vi "SerialPositionCalibration.vi"() -> ()   [LabVIEW 2017]
uses:
  <vilib>/Analysis/baseanly.llb/Mean (DBL).vi
  <vilib>/Instr/_visa.llb/VISA Configure Serial Port (Instr).vi
  <vilib>/express/express shared/transition.llb/Dynamic To Waveform Array.vi
  <vilib>/express/express signal manip/GetorSetDDTAttributes/Set DDT Attributes/SetT0.vi
  <vilib>/express/express shared/transition.llb/Waveform Array To Dynamic.vi
  <vilib>/express/express signal manip/GetorSetDDTAttributes/Set DDT Attributes/Set DDT Properties.xnode
  <vilib>/Analysis/NI_AALBase.lvlib
  <vilib>/Analysis/NI_AALPro.lvlib
panel:
  in  "Filename":path=path "Servo1PosCal.xlsx"
  out "PWM Array":dbl[](array[numeric])
  out "Angle vs PWM Quadratic Coefficients":dbl[](array[numeric])
  out "Angle vs PWM Linear Coefficients":dbl[](array[numeric])
  out "Angle vs PWM":cluster{dbl[], dbl[]}(graph)
  out "ADC vs  Angle Quadratic Coefficients":dbl[](array[numeric])
  out "ADC vs  Angle Linear Coefficients":dbl[](array[numeric])
  in  "Save Data":bool
  in  "Baud Rate":dbl=115200.0
  out "Angle Array":dbl[](array[numeric])
  out "ADC Value Array":dbl[](array[numeric])
  out "ADC Value vs Angle":cluster{dbl[], dbl[]}(graph)
  out "Average ADC Value":dbl format="%0.2f"
  out "Live ADC Value":cluster{i32, dbl, dbl[]}(graph)
  in  "Com Port":refnum<visa-resource-name>="ASRL1::INSTR"
  in  "Sample Frequency":dbl=200.0
  in  "Number of Samples":dbl=100.0
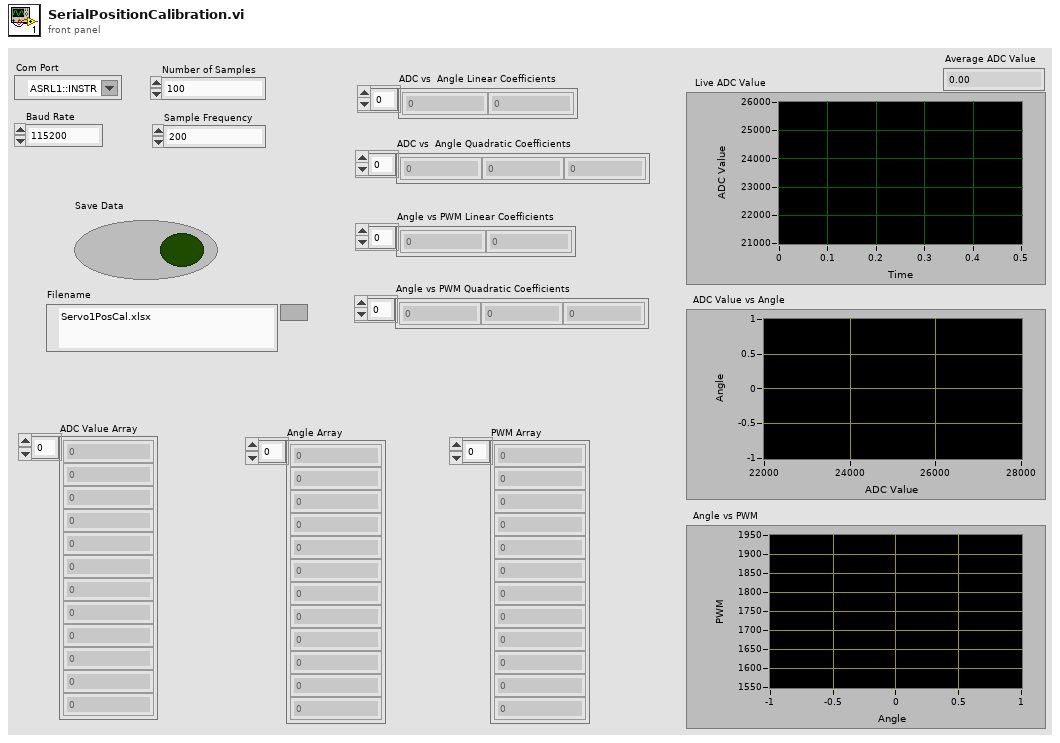
[diagram p1: front panel]
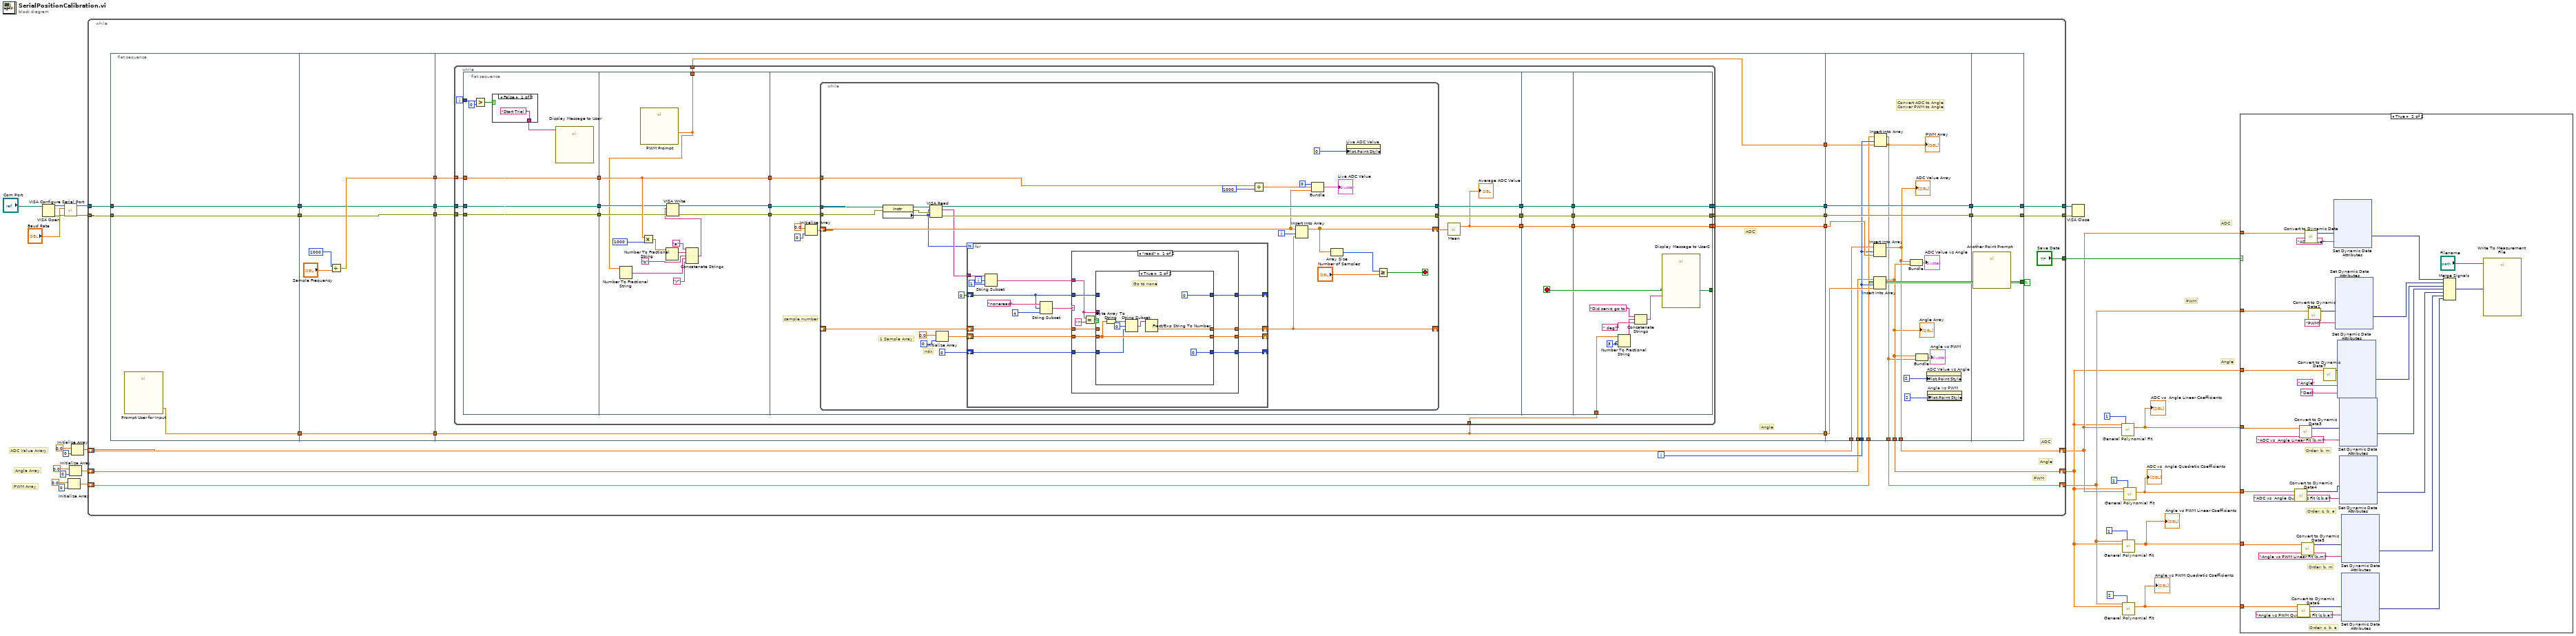
[diagram p0: block diagram]
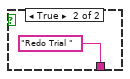
[diagram p3: hidden frame]
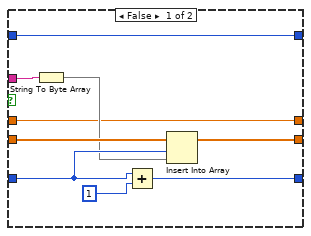
[diagram p4: hidden frame]
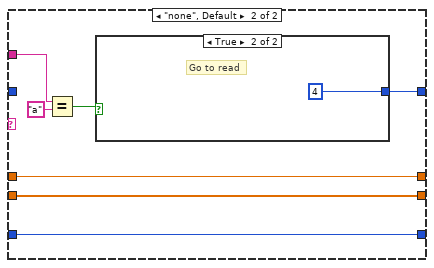
[diagram p5: hidden frame]
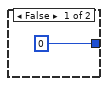
[diagram p6: hidden frame]
diagram:
  # "PWM Array"
  # "ADC"
  # "PWM"
  # "Angle"
  # "Angle Array"
  # "ADC Value Arrary"
  n1 = VISA Open(VISA resource name="Com Port") -> (VISA resource name=w28:refnum<visa-resource-name>, error out=w27:errorcluster)  [unwired: 4 in]
  n2 = call-poly "VISA Configure Serial Port"("VISA resource name"=w28, "baud rate (9600)"="Baud Rate", "error in (no error)"=w27) -> ("VISA resource name out"=w26:refnum<visa-resource-name>, "error out"=w25:errorcluster)  [unwired: 11 in]
  n3 = Initialize Array(0.0 ("element"), 0 ("dimension size")) -> (w4:dbl[])
  n4 = Initialize Array(0.0 ("element"), 0 ("dimension size")) -> (w17:dbl[])
  n5 = Initialize Array(0.0 ("element"), 0 ("dimension size")) -> (w18:dbl[])
  n6 = while {
    tunnel: w26 -> [w55]
    tunnel: w25 -> [w54]
    tunnel: [w52] -> w24
    tunnel: [w51] -> w23
    shift-right: [w32] -> w2
    shift-left: w18 -> [w35]
    shift-right: [w33] -> w1
    shift-left: w17 -> [w34]
    tunnel: ["Save Data"] -> w15
    shift-right: [w30] -> w3
    shift-left: w4 -> [w31]
    i -> [w40]
    stop <- w56 continue-if-true
    # "PWM"
    # "Angle"
    # "ADC"
    n7 = flat-sequence {
      tunnel: w54 -> [w58]
      tunnel: w55 -> [w59]
      tunnel: [w59] -> w49
      tunnel: [w58] -> w48
      tunnel: [w57] -> w46
      tunnel: [w60] -> w53
      tunnel: [w62] -> w50
      tunnel: w49 -> [w61]
      tunnel: w48 -> [w60]
      tunnel: [w64] -> w47
      tunnel: w46 -> [w64]
      tunnel: [w61] -> w45
      tunnel: w53 -> [w72]
      tunnel: [w68] -> w43
      tunnel: w50 -> [w71]
      tunnel: w47 -> [w67]
      tunnel: w45 -> [w73]
      tunnel: [w67] -> w39
      tunnel: [w70] -> w38
      tunnel: [w69] -> w37
      tunnel: [w66] -> w36
      tunnel: w43 -> [w236]
      tunnel: [w236] -> w42
      tunnel: [w235] -> w41
      tunnel: w40 -> [w228]
      tunnel: w39 -> [w232]
      tunnel: w38 -> [w229]
      tunnel: w37 -> [w235]
      tunnel: w36 -> [w227]
      tunnel: w35 -> [w226]
      tunnel: w34 -> [w225]
      tunnel: [w222] -> w33
      tunnel: [w224] -> w32
      tunnel: w31 -> [w223]
      tunnel: [w221] -> w30
      tunnel: [w239] -> w56
      tunnel: w42 -> [w238]
      tunnel: [w238] -> w52
      tunnel: [w237] -> w51
      tunnel: w41 -> [w237]
      frame #0 {
        n8 = call "Prompt User for Input"() -> ("Angle"=w57:dbl)  [unwired: 17 in, 2 out]
      }
      frame #1 {
        n9 = Divide(x=1000, y="Sample Frequency") -> (x/y=w62:dbl)
      }
      frame #2 {
        # "Angle"
        # "ADC"
        n10 = while {
          tunnel: w73 -> [w94]
          tunnel: w72 -> [w93]
          tunnel: [w92] -> w68
          tunnel: [w91] -> w69
          tunnel: w71 -> [w90]
          tunnel: [w89] -> w70
          tunnel: w67 -> [w81]
          tunnel: [w74] -> w66
          i -> [w82]
          stop <- w95 stop-if-true
          n11 = flat-sequence {
            tunnel: w90 -> [w100]
            tunnel: w93 -> [w101]
            tunnel: w94 -> [w102]
            tunnel: [w102] -> w80
            tunnel: [w101] -> w78
            tunnel: [w100] -> w77
            tunnel: w82 -> [w99]
            tunnel: w80 -> [w110]
            tunnel: [w108] -> w79
            tunnel: w78 -> [w109]
            tunnel: w77 -> [w111]
            tunnel: [w111] -> w76
            tunnel: [w107] -> w75
            tunnel: [w106] -> w74
            tunnel: [w126] -> w88
            tunnel: [w125] -> w86
            tunnel: [w119] -> w84
            tunnel: w79 -> [w128]
            tunnel: w76 -> [w124]
            tunnel: w75 -> [w127]
            tunnel: w88 -> [w210]
            tunnel: [w210] -> w87
            tunnel: w86 -> [w209]
            tunnel: [w209] -> w85
            tunnel: w84 -> [w208]
            tunnel: [w208] -> w83
            tunnel: [w217] -> w95
            tunnel: w87 -> [w220]
            tunnel: [w220] -> w92
            tunnel: [w219] -> w91
            tunnel: w85 -> [w219]
            tunnel: w83 -> [w218]
            tunnel: [w218] -> w89
            tunnel: w81 -> [w213]
            frame #0 {
              n12 = Greater?(x=w99, y=0) -> (0:w98:bool)
              n13 = case shown="False" w98 {
                tunnel: ["Start Trial " ("Message") "Redo Trial " ("Message")] -> w96
                frame False {
                }
                frame True {
                }
              }
              n14 = call "Display Message to User"("Message"=w96) -> ()  [unwired: 9 in, 2 out]
            }
            frame #1 {
              n15 = call "PWM Prompt"() -> ("PWM"=w106:dbl)  [unwired: 17 in, 2 out]
              n16 = Number To Fractional String(number=w106) -> (F-format string=w117:string)  [unwired: 3 in]
              n17 = Multiply(x=w111, y=1000) -> (x*y=w118:dbl)
              n18 = Number To Fractional String(number=w118) -> (F-format string=w116:string)  [unwired: 3 in]
              n19 = Concatenate Strings("a", w116, "b", w117, "\r") -> (w105:string)
              n20 = VISA Write(VISA resource name=w110, write buffer=w105, error in (no error)=w109) -> (VISA resource name out=w108:refnum<visa-resource-name>, error out=w107:errorcluster)  [unwired: 1 out]
            }
            frame #2 {
              # "sample number"
              n21 = Initialize Array(0.0, 0 ("dimension size")) -> (w123:dbl[])
              n22 = while {
                tunnel: w128 -> [w153]
                tunnel: w127 -> [w152]
                tunnel: [w151] -> w126
                tunnel: [w150] -> w125
                shift-right: [w138] -> _
                shift-left: _ -> [w144]
                tunnel: w124 -> [w133]
                shift-right: [w136] -> w120
                shift-left: w123 -> [w137]
                i -> [w139]
                stop <- w142 stop-if-true
                # "ndx"
                # "1 Sample Array"
                n23 = property class="Instr"(reference=w153, error in=w152) -> (reference out=w155:refnum<visa-resource-name>, error out=w154:errorcluster, "Serial Settings:Number of Bytes at Serial Port"=w130:u32)
                n24 = VISA Read(VISA resource name=w155, byte count=w130, error in (no error)=w154) -> (VISA resource name out=w151:refnum<visa-resource-name>, read buffer=w131:string, error out=w150:errorcluster)  [unwired: 1 out]
                n25 = Initialize Array(0.0 ("element"), 0 ("dimension size")) -> (w146:dbl[])
                n26 = for {
                  N: w130 -> [_]
                  tunnel: w131 -> [w169]
                  shift-right: [w165] -> _
                  shift-left: 0 -> [w164]
                  shift-right: [w160] -> _
                  shift-left: w146 -> [w161]
                  shift-right: [w159] -> _
                  shift-left: 0 ("dimension size") -> [w162]
                  shift-right: [w158] -> w138
                  shift-left: w144 -> [w157]
                  i -> [w168]
                  n27 = String Subset(string=w169, offset (0)=w168, length (rest)=1 ("length (rest)")) -> (substring=w163:string)
                  n28 = String Subset(string="noneread", offset (0)=w164, length (rest)=4 ("length (rest)")) -> (substring=w156:string)
                  n29 = case shown="\"read\"" w156 {
                    tunnel: [w181 w203] -> w165
                    tunnel: w164 -> [w180 _]
                    tunnel: w163 -> [w177 w202]
                    tunnel: w162 -> [w176 w199]
                    tunnel: w161 -> [w175 w200]
                    tunnel: [w174 w200] -> w160
                    tunnel: [w173 w199] -> w159
                    tunnel: [w172 w201] -> w158
                    tunnel: w157 -> [w171 w201]
                    frame "read" {
                      n30 = Equal?(x=w177, y="!") -> (x = y?=w179:bool)
                      n31 = case shown="True" w179 {
                        tunnel: [w190 0] -> w181
                        tunnel: w180 -> [w190 _]
                        tunnel: w177 -> [w187 _]
                        tunnel: w176 -> [w188 w192]
                        tunnel: w175 -> [w189 w195]
                        tunnel: [w185 w195] -> w174
                        tunnel: [w184 0] -> w173
                        tunnel: [w183 w197] -> w172
                        tunnel: w171 -> [w183 _]
                        frame False {
                          n32 = String To Byte Array(string=w187) -> (unsigned byte array=w186:u8[])
                          n33 = Add(x=w188, y=1 ("dimension size")) -> (x+y=w184:i32)
                          n34 = Insert Into Array(array=w189, index=w188, new element=w186) -> (w185:dbl[])
                        }
                        frame True {
                          # "Go to none"
                          n35 = Byte Array To String(unsigned byte array=w195) -> (string=w194:string)
                          n36 = String Subset(string=w194, offset (0)=0, length (rest)=w192) -> (substring=w193:string)
                          n37 = Fract/Exp String To Number(string=w193) -> (number=w197:dbl)  [unwired: 3 in, 1 out]
                        }
                      }
                    }
                    frame "none", Default {
                      n38 = Equal?(x=w202, y="a") -> (x = y?=w205:bool)
                      n39 = case shown="True" w205 {
                        tunnel: [0 4] -> w203
                        frame False {
                        }
                        frame True {
                          # "Go to read"
                        }
                      }
                    }
                  }
                }
                n40 = Divide(x=w133, y=1000) -> (x/y=w132:dbl)
                n41 = Insert Into Array(array=w137, index=w139, new element=w138) -> (w136:dbl[])
                n42 = Bundle(0, w132, w137) -> (→"Live ADC Value":cluster{i32, dbl, dbl[]})  [unwired: 1 in]
                n43 = Array Size(array=w136) -> (size(s)=w135:i32)
                n44 = property on="Live ADC Value" class="WFGraph (strict)"("Plot.Point Style"=u8 0) -> ()  [unwired: 2 in, 2 out]
                n45 = Greater Or Equal?(x=w135, y="Number of Samples") -> (x >= y?=w142:bool)
              }
              n46 = call-poly <vilib>:"Mean.vi"("X"=w120) -> ("mean"=w119:dbl)  [unwired: 1 out]
              "Average ADC Value" <- w119
            }
            frame #3 {
            }
            frame #4 {
              w211 = 3
              n47 = Number To Fractional String(number=w213, width (-)=w211, precision (6)=w211) -> (F-format string=w214:string)  [unwired: 1 in]
              n48 = Concatenate Strings("Did servo go to ", w214, " deg?") -> (w212:string)
              n49 = call "Display Message to User2"("Message"=w212) -> ("Yes"=w217:bool)  [unwired: 9 in, 1 out]
            }
          }
        }
      }
      frame #3 {
        # "Convert ADC to Angle\nConver PWM to Angle"
        n50 = Insert Into Array(array=w226, index=w228, new element=w229) -> (w224:dbl[])
        "ADC Value Array" <- w224
        n51 = Insert Into Array(array=w225, index=w228, new element=w232) -> (w222:dbl[])
        "Angle Array" <- w222
        n52 = Insert Into Array(array=w223, index=w228, new element=w227) -> (w221:dbl[])
        "PWM Array" <- w221
        n53 = Bundle(w224, w222) -> (→"ADC Value vs Angle":cluster{dbl[], dbl[]})  [unwired: 1 in]
        n54 = Bundle(w222, w221) -> (→"Angle vs PWM":cluster{dbl[], dbl[]})  [unwired: 1 in]
        n55 = property on="ADC Value vs Angle" class="XYGraph (strict)"("Plot.Point Style"=u8 2) -> ()  [unwired: 2 in, 2 out]
        n56 = property on="Angle vs PWM" class="XYGraph (strict)"("Plot.Point Style"=u8 2) -> ()  [unwired: 2 in, 2 out]
      }
      frame #4 {
        n57 = call "Another Point Prompt"() -> ("OK"=w239:bool)  [unwired: 18 in, 1 out]
      }
    }
  }
  n58 = VISA Close(VISA resource name=w24, error in (no error)=w23) -> ()  [unwired: 1 out]
  n59 = call <vilib>:"General Polynomial Fit.vi"("Y"=w1, "polynomial order"=1, "X"=w2) -> ("Polynomial Coefficients"=w12:dbl[])  [unwired: 9 in, 3 out]
  "ADC vs  Angle Linear Coefficients" <- w12
  n60 = call <vilib>:"General Polynomial Fit.vi"("Y"=w3, "polynomial order"=1, "X"=w1) -> ("Polynomial Coefficients"=w7:dbl[])  [unwired: 9 in, 3 out]
  "Angle vs PWM Linear Coefficients" <- w7
  n61 = call <vilib>:"General Polynomial Fit.vi"("Y"=w3, "polynomial order"=2, "X"=w1) -> ("Polynomial Coefficients"=w8:dbl[])  [unwired: 9 in, 3 out]
  "Angle vs PWM Quadratic Coefficients" <- w8
  n62 = call <vilib>:"General Polynomial Fit.vi"("Y"=w1, "polynomial order"=2, "X"=w2) -> ("Polynomial Coefficients"=w11:dbl[])  [unwired: 9 in, 3 out]
  "ADC vs  Angle Quadratic Coefficients" <- w11
  n63 = case shown="True" w15 {
    tunnel: w2 -> [_ w270]
    tunnel: w3 -> [_ w267]
    tunnel: w12 -> [_ w264]
    tunnel: w11 -> [_ w263]
    tunnel: w7 -> [_ w252]
    tunnel: w8 -> [_ w251]
    tunnel: w1 -> [_ w250]
    frame False {
    }
    frame True {
      # "Order: c, b, a"
      # "Order: b, m"
      # "Order: c, b, a"
      # "Order: b, m"
      n64 = call "Convert to Dynamic Data4"("Array"=w263) -> ("Dynamic Data Type"=w240:dynamicdata)  [unwired: 3 in]
      n65 = call "Convert to Dynamic Data6"("Array"=w251) -> ("Dynamic Data Type"=w255:dynamicdata)  [unwired: 3 in]
      n66 = call "Convert to Dynamic Data3"("Array"=w264) -> ("Dynamic Data Type"=w262:dynamicdata)  [unwired: 3 in]
      n67 = call "Convert to Dynamic Data5"("Array"=w252) -> ("Dynamic Data Type"=w256:dynamicdata)  [unwired: 3 in]
      n68 = call "Convert to Dynamic Data"("Array"=w270) -> ("Dynamic Data Type"=w269:dynamicdata)  [unwired: 3 in]
      n69 = call "Convert to Dynamic Data2"("Array"=w267) -> ("Dynamic Data Type"=w266:dynamicdata)  [unwired: 3 in]
      n70 = call "Convert to Dynamic Data7"("Array"=w250) -> ("Dynamic Data Type"=w249:dynamicdata)  [unwired: 3 in]
      n71 = xnode "Set Dynamic Data Attributes"("Signals In"=w269, "Signal Name"="ADC Value") -> ("Signals Out"=w259:dynamicdata)  [unwired: 2 in, 1 out]
      n72 = xnode "Set Dynamic Data Attributes"("Signals In"=w266, "Signal Name"="PWM") -> ("Signals Out"=w258:dynamicdata)  [unwired: 3 in, 1 out]
      n73 = xnode "Set Dynamic Data Attributes"("Signals In"=w249, "Signal Name"="Angle", "Unit"="Ded" ("Signal Name")) -> ("Signals Out"=w244:dynamicdata)  [unwired: 2 in, 1 out]
      n74 = xnode "Set Dynamic Data Attributes"("Signals In"=w262, "Signal Name"="ADC vs  Angle Linear Fit (b,m)") -> ("Signals Out"=w245:dynamicdata)  [unwired: 2 in, 1 out]
      n75 = xnode "Set Dynamic Data Attributes"("Signals In"=w240, "Signal Name"="ADC vs  Angle Quadratic Fit (c,b,a)") -> ("Signals Out"=w246:dynamicdata)  [unwired: 2 in, 1 out]
      n76 = xnode "Set Dynamic Data Attributes"("Signals In"=w256, "Signal Name"="Angle vs PWM Linear Fit (b,m)") -> ("Signals Out"=w243:dynamicdata)  [unwired: 2 in, 1 out]
      n77 = xnode "Set Dynamic Data Attributes"("Signals In"=w255, "Signal Name"="Angle vs PWM Quadratic Fit (c,b,a)") -> ("Signals Out"=w242:dynamicdata)  [unwired: 2 in, 1 out]
      n78 = Merge Signals(w259, w258, w244, w245, w246, w243, w242) -> (w257:dynamicdata)
      n79 = call "Write To Measurement File"("Signals"=w257, "Filename"="Filename") -> ()  [unwired: 15 in, 3 out]
    }
  }
